vi "Select and Initiate Script.vi"(8 "error in (no error)":errorcluster, 10 "script name":string, 11 "Semiconductor Module Context":T1) -> (0 "error out":errorcluster, 2 "HSDIO GEN Sessions Out":refnum<k15>[](array[refnum]), 3 "Semiconductor Module Context Out":T1)   [LabVIEW 2013]
doc: "Selects and initiates the script name selected."
uses:
  <vilib>/NI_TestStand_SemiconductorModule/NI_TestStand_Semiconductor_Module.lvlibp/PinMap/General/SemiconductorModuleContext.ctl
  <vilib>/NI_TestStand_SemiconductorModule/NI_TestStand_Semiconductor_Module.lvlibp
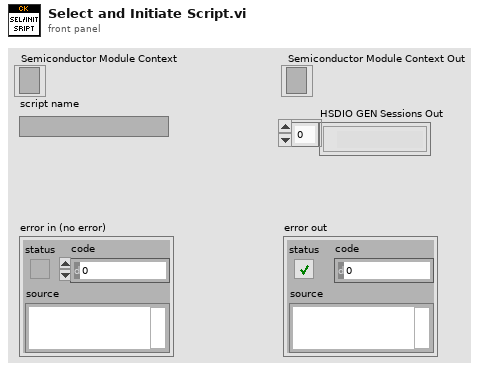
[diagram p1: front panel]
types:
  T1 = typedef "NI_TestStand_Semiconductor_Module.lvlibp/SemiconductorModuleContext.ctl" = refnum<k7>
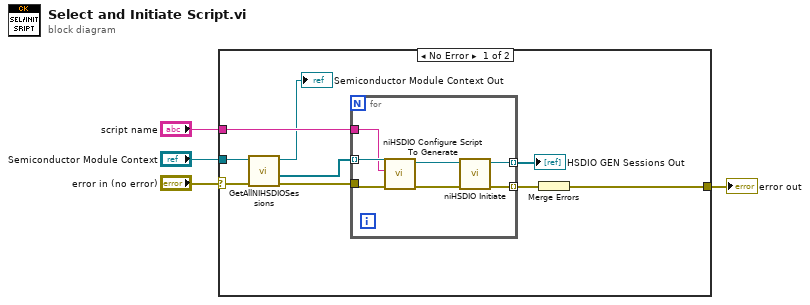
[diagram p0: block diagram]
diagram:
  n1 = case shown="No Error" "error in (no error)" {
    selector: "error in (no error)" -> [w8 w21]
    tunnel: "Semiconductor Module Context" -> [w13 _]
    tunnel: "script name" -> [w11 _]
    tunnel: [w9 w21] -> w2
    frame No Error {
      n2 = call <vilib>:"GetAllNIHSDIOSessions.vi"("error in (no error)"=w8, "Semiconductor Module Context"=w13) -> ("error out"=w7:errorcluster, "Generation Sessions"=w12:refnum<k15>[], "Semiconductor Module Context Out"=→"Semiconductor Module Context Out":T1)  [unwired: 6 in, 1 out]
      n3 = for {
        tunnel: w7 -> [w15]
        tunnel: w12 -> [w20] mode=indexing
        tunnel: w11 -> [w19]
        tunnel: [w17] -> w10 mode=indexing
        tunnel: [w16] -> w5 mode=indexing
        n4 = call <instrlib>:"niHSDIO Configure Script To Generate.vi"("error in (no error)"=w15, "script name"=w19, "instrument handle"=w20) -> ("error out"=w14:errorcluster, "instrument handle out"=w18:refnum<k15>)  [unwired: 7 in]
        n5 = call <instrlib>:"niHSDIO Initiate.vi"("error in (no error)"=w14, "instrument handle"=w18) -> ("error out"=w17:errorcluster, "instrument handle out"=w16:refnum<k15>)  [unwired: 8 in]
      }
      "HSDIO GEN Sessions Out" <- w5
      n6 = Merge Errors(w10) -> (w9:errorcluster)
    }
    frame Error {
    }
  }
  "error out" <- w2
